vi "Acquire_OSCILL_SubVI_v2.vi"(4 "mV/div [CH2]":dbl=520.0, 6 "Vertical Offset CH1":dbl, 7 "Vertical Offset CH2":dbl=1.5 format="%#_13g", 8 "error in (no error)":errorcluster, 9 "mV/div [CH1]":dbl=5.0, 10 "N_acquisition":i32, 11 "VISA resource name":refnum<visa-resource-name>) -> (0 "error out":errorcluster, 1 "Time":dbl[](array[numeric]), 2 "CH2_averaged":dbl[](array[numeric]), 3 "CH1_averaged":dbl[](array[numeric]), 5 "VISA resource name out":refnum<visa-resource-name>)   [LabVIEW 2017]
uses:
  Agilent 2000 3000 X-Series/Agilent 2000 3000 X-Series.lvlib
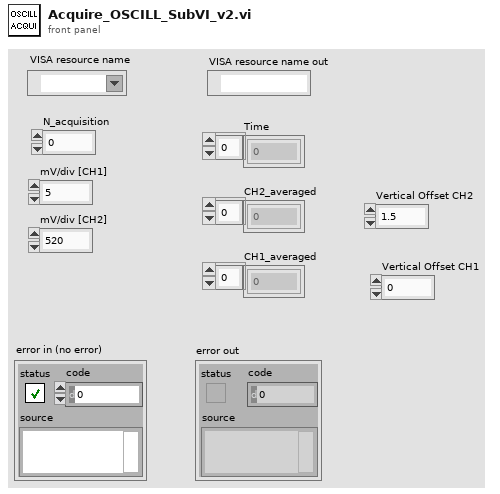
[diagram p1: front panel]
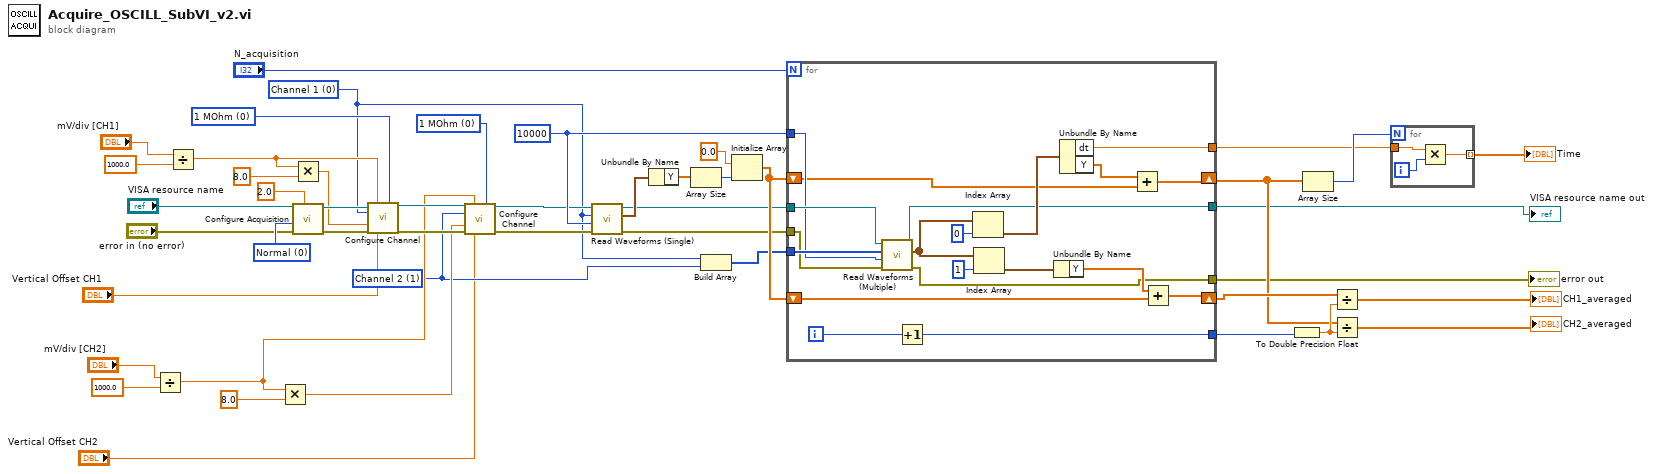
[diagram p0: block diagram]
diagram:
  w4 = 0 items=["Channel 1", "Channel 2", "Channel 3", "Channel 4"] ("Channel Name (0: Channel 1)")
  w5 = 1 items=["Channel 1", "Channel 2", "Channel 3", "Channel 4"] ("Channel Name (0: Channel 1)")
  w6 = 0 items=["1 MOhm", "50 Ohm"] ("Impedance (0: 1 MOhm)")
  w8 = 0 items=["1 MOhm", "50 Ohm"] ("Impedance (0: 1 MOhm)")
  w45 = 0 items=["Normal", "Average", "High Resolution", "Peak"] ("Acquisition Type (0: Normal)")
  w46 = u32 10000 ("y")
  n1 = Divide(x="mV/div [CH2]", y=1000.0) -> (x/y=w9:dbl)
  n2 = Divide(x="mV/div [CH1]", y=1000.0) -> (x/y=w36:dbl)
  n3 = Multiply(x=w9, y=8.0) -> (x*y=w10:dbl)
  n4 = Multiply(x=w36, y=8.0) -> (x*y=w18:dbl)
  n5 = call "Configure Acquisition.vi"("Average Count (8)"=2.0, "error in (no error)"="error in (no error)", "Acquisition Type (0: Normal)"=w45, "VISA resource name"="VISA resource name") -> ("error out"=w39:errorcluster, "VISA resource name out"=w40:refnum<visa-resource-name>)  [unwired: 6 in]
  n6 = call "Configure Channel.vi"("VISA resource name"=w40, "Vertical Scale (5.0 V)"=w36, "Impedance (0: 1 MOhm)"=w8, "Channel Name (0: Channel 1)"=w4, "Vertical Range (40.0 V)"=w18, "error in (no error)"=w39, "Vertical Offset (0.0)"="Vertical Offset CH1") -> ("VISA resource name out"=w15:refnum<visa-resource-name>, "error out"=w12:errorcluster)  [unwired: 4 in, 3 out]
  n7 = call "Configure Channel.vi"("VISA resource name"=w15, "Vertical Scale (5.0 V)"=w9, "Impedance (0: 1 MOhm)"=w6, "Channel Name (0: Channel 1)"=w5, "Vertical Range (40.0 V)"=w10, "error in (no error)"=w12, "Vertical Offset (0.0)"="Vertical Offset CH2") -> ("VISA resource name out"=w14:refnum<visa-resource-name>, "error out"=w13:errorcluster)  [unwired: 4 in, 3 out]
  n8 = call "Read Waveforms (Single).vi"("error in (no error)"=w13, "Timeout (10000 ms)"=w46, "Source Channel (0: Channel 1)"=w4, "VISA resource name"=w14) -> ("error out"=w34:errorcluster, "Waveform Data"=w42:waveform(dbl), "VISA resource name out"=w33:refnum<visa-resource-name>)  [unwired: 1 in, 4 out]
  n9 = Unbundle By Name(w42) -> ("Y"=w43:dbl[])
  n10 = Array Size(array=w43) -> (size(s)=w44:i32)
  n11 = Build Array(w4, w5) -> (w30:i32[])
  n12 = Initialize Array(0.0 ("element"), w44) -> (w47:dbl[])
  n13 = for {
    N: "N_acquisition" -> [_]
    tunnel: w46 -> [w65]
    shift-right: [w57] -> w23
    shift-left: w47 -> [w55]
    tunnel: [w48] -> w25
    shift-right: [w53] -> w24
    shift-left: w47 -> [w52]
    tunnel: w34 -> [w64]
    tunnel: w33 -> [w67]
    tunnel: w30 -> [w66]
    tunnel: [w58] -> w28
    tunnel: [w51] -> w20
    tunnel: [w50] -> w19
    i -> [w49]
    n14 = call "Read Waveforms (Multiple).vi"("error in (no error)"=w64, "Timeout (10000 ms)"=w65, "Channels"=w66, "VISA resource name"=w67) -> ("error out"=w50:errorcluster, "Waveform Data"=w61:waveform(dbl)[], "VISA resource name out"=w51:refnum<visa-resource-name>)  [unwired: 5 out]
    n15 = Increment(x=w49) -> (x+1=w48:i32)
    n16 = Index Array(array=w61, index=0) -> (element=w59:waveform(dbl))
    n17 = Index Array(array=w61, index=1) -> (element=w60:waveform(dbl))
    n18 = Unbundle By Name(w60) -> ("Y"=w54:dbl[])
    n19 = Unbundle By Name(w59) -> ("dt"=w58:dbl, "Y"=w56:dbl[])
    n20 = Add(x=w56, y=w55) -> (x+y=w57:dbl[])
    n21 = Add(x=w54, y=w52) -> (x+y=w53:dbl[])
  }
  "error out" <- w19
  "VISA resource name out" <- w20
  n22 = To Double Precision Float(number=w25) -> (double precision float=w26:dbl)
  n23 = Array Size(array=w23) -> (size(s)=w29:i32)
  n24 = Divide(x=w24, y=w26) -> (x/y=→"CH1_averaged":dbl[])
  n25 = Divide(x=w23, y=w26) -> (x/y=→"CH2_averaged":dbl[])
  n26 = for {
    N: w29 -> [_]
    tunnel: w28 -> [w69]
    tunnel: [w70] -> w27 mode=indexing
    i -> [w68]
    n27 = Multiply(x=w69, y=w68) -> (x*y=w70:dbl)
  }
  "Time" <- w27
